vi "Initialize.vi"(4 "stop bits (1.0)":u16(ring)=10 items=["1.0"=10, "1.5"=15, "2.0"=20], 6 "parity (none)":u16(ring) items=["None", "Odd", "Even", "Mark", "Space"], 8 "error in (no error)":errorcluster, 9 "data bits (8)":u16=8, 10 "baud rate (9600)":u32=9600, 11 "port":refnum<visa-resource-name>) -> (0 "error out":errorcluster, 3 "Comdel out":refnum<class "PL Comdel CX.lvclass">)   [LabVIEW 2015, in "PL Comdel CX.lvclass"]
doc: "Initializes connection to device using specified settings."
uses:
  PL Comdel CX.lvclass
  PL Comdel CX.lvclass/PL Comdel CX.ctl
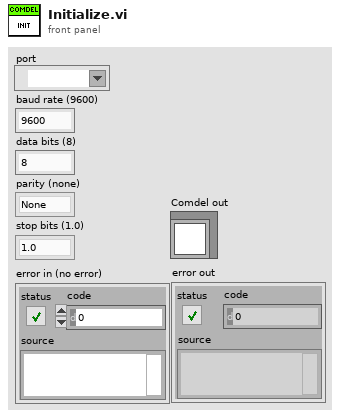
[diagram p1: front panel]
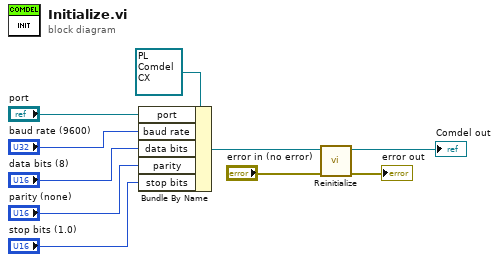
[diagram p0: block diagram]
diagram:
  n1 = Bundle By Name(cluster=refnum<class "PL Comdel CX.lvclass"> refnum ("PL Comdel CX.lvclass"), "port"="port", "baud rate"="baud rate (9600)", "data bits"="data bits (8)", "parity"="parity (none)", "stop bits"="stop bits (1.0)") -> (w10:refnum<class "PL Comdel CX.lvclass">)
  n2 = call "Reinitialize.vi"("error in (no error)"="error in (no error)", "Comdel in"=w10) -> ("error out"=→"error out":errorcluster, "Comdel out"=→"Comdel out":refnum<class "PL Comdel CX.lvclass">)  [unwired: 8 in]
